vi "dfd_Maxflat Param Validation.vi"(6 "fs":dbl=1.0, 7 "symmetric FIR ? (T)":bool, 8 "error in (no error)":errorcluster, 9 "3dB cutoff freq":dbl=0.25, 10 "denominator order":i32=2, 11 "numerator order":i32=2) -> (0 "error out":errorcluster, 1 "normalized fc":dbl=0.2, 2 "dup denominator order":i32, 3 "mod numerator order":i32=2, 5 "symmetric FIR out":bool)   [LabVIEW 2017, in "NI_DigFilter_Design.lvlib"]
doc: "Validates the input parameters of the Maxflat filter design."
uses:
  <vilib>/addons/Digital Filter Design/NI_DigFilter_Design.lvlib
  <vilib>/addons/Digital Filter Design/_Misc.llb/dfd_Error Handlers (Multiple).vi
  <vilib>/addons/Digital Filter Design/NI_DigFilterLicensed.lvlib
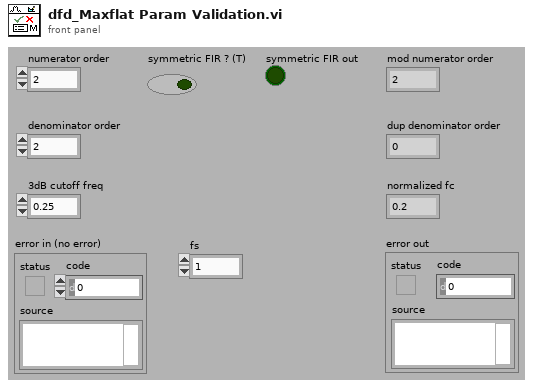
[diagram p1: front panel]
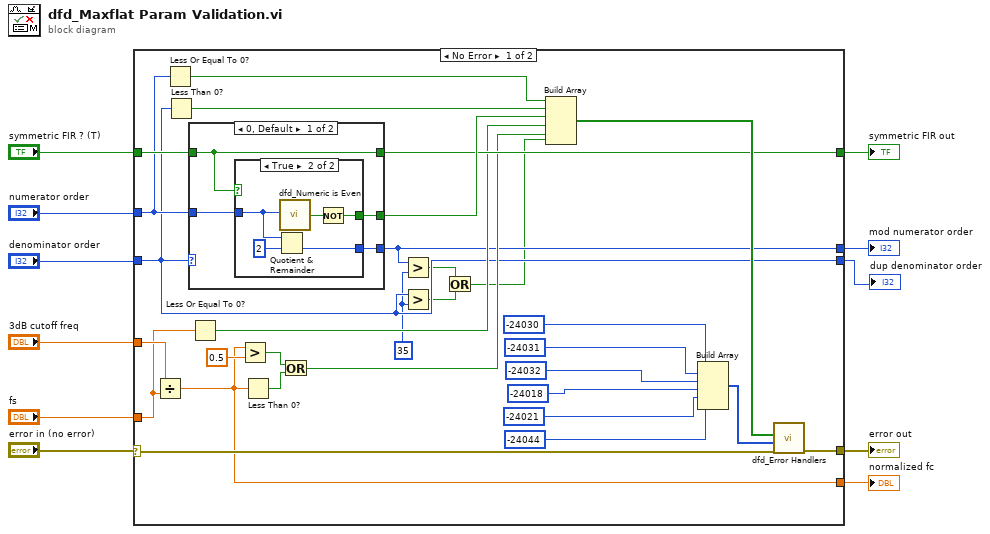
[diagram p0: block diagram]
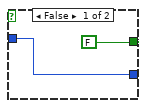
[diagram p2: hidden frame]
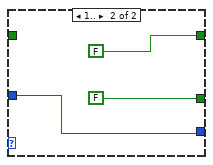
[diagram p3: hidden frame]
diagram:
  n1 = case shown="No Error" "error in (no error)" {
    selector: "error in (no error)" -> [w31 w56]
    tunnel: "denominator order" -> [w17 _]
    tunnel: "symmetric FIR ? (T)" -> [w41 _]
    tunnel: "numerator order" -> [w40 _]
    tunnel: [w30 w56] -> w7
    tunnel: "3dB cutoff freq" -> [w29 _]
    tunnel: "fs" -> [w26 _]
    tunnel: [w18 _] -> w4
    tunnel: [w27 _] -> w3
    tunnel: [w25 _] -> w2
    tunnel: [w17 _] -> w1
    frame No Error {
      w16 = 35 ("y")
      n2 = Divide(x=w29, y=w26) -> (x/y=w25:dbl)
      n3 = Less Or Equal To 0?(x=w40) -> (x <= 0?=w38:bool)
      n4 = Less Than 0?(x=w17) -> (x < 0?=w39:bool)
      n5 = case shown="0, Default" w17 {
        tunnel: w41 -> [w42 _]
        tunnel: w40 -> [w45 w54]
        tunnel: [w44 FALSE] -> w37
        tunnel: [w43 w54] -> w18
        tunnel: [w42 FALSE] -> w27
        frame 0, Default {
          n6 = case shown="True" w42 {
            tunnel: w45 -> [w46 w50]
            tunnel: [FALSE w51] -> w44
            tunnel: [w46 w48] -> w43
            frame False {
            }
            frame True {
              n7 = Quotient & Remainder(x=w50, y=2) -> (floor(x/y)=w48:i32)  [unwired: 1 out]
              n8 = call <vilib>:"dfd_Numeric is Even.vi"("N"=w50) -> ("even ?"=w52:bool)
              n9 = Not(x=w52) -> (.not. x?=w51:bool)
            }
          }
        }
        frame 1.. {
        }
      }
      n10 = Less Or Equal To 0?(x=w26) -> (x <= 0?=w19:bool)
      n11 = Greater?(x=w25, y=0.5) -> (0:w22:bool)
      n12 = Less Than 0?(x=w25) -> (x < 0?=w21:bool)
      n13 = Or(x=w22, y=w21) -> (x .or. y?=w20:bool)
      n14 = Greater?(x=w18, y=w16) -> (0:w15:bool)
      n15 = Greater?(x=w17, y=w16) -> (0:w14:bool)
      n16 = Or(x=w15, y=w14) -> (x .or. y?=w13:bool)
      n17 = Build Array(w38, w39, w37, w19, w20, w13) -> (w32:bool[])
      n18 = Build Array(-24030 ("ERR_ORDER_NUM_LE_ZERO"), -24031 ("ERR_ORDER_DEN_LT_ZERO"), -24032 ("ERR_ORDER_ODD"), -24018 ("ERR_FS_LE_ZERO"), -24021 ("ERR_FREQ_RANGE_WRONG"), -24044 ("ERR_ORDER_TOO_HIGH")) -> (w33:i32[])
      n19 = call-poly <vilib>:"dfd_Error Handlers.vi"("error in (no error)"=w31, "error sources"=w33, "condition failed?"=w32) -> ("error out"=w30:errorcluster)  [unwired: 8 out]
    }
    frame Error {
    }
  }
  "error out" <- w7
  "mod numerator order" <- w4
  "symmetric FIR out" <- w3
  "normalized fc" <- w2
  "dup denominator order" <- w1
